vi "Read Joystick.vi"   [LabVIEW 2020]
uses:
  <vilib>/Rock Robotics/WPI/Utilities/WPI_GetSetVariantRefNum.vi
  <vilib>/Rock Robotics/Network Tables/NT Write Boolean Array.vi
  <vilib>/Rock Robotics/Network Tables/NT Write Numeric Array.vi
  Robot Global Data.vi
types:
  T1 = typedef "WPI_JoystickDevRef.ctl" = cluster{"Device":T2}
  T2 = typedef "WPI_JoystickDeviceEnum.ctl" = enum16{"USB 0", "USB 1", "USB 2", "USB 3", "USB 4", "USB 5"}
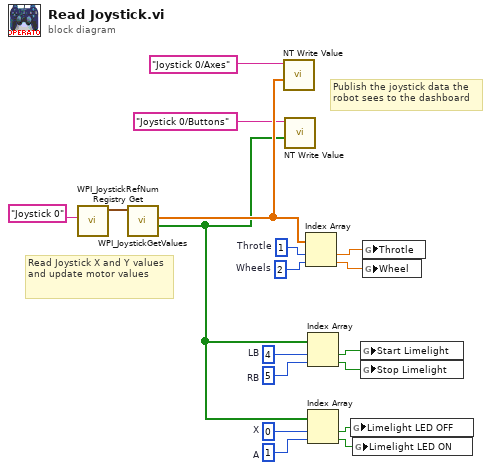
[diagram p0: block diagram]
diagram:
  w3 = 1  # A
  w2 = 0  # X
  w8 = 5  # RB
  w18 = 4  # LB
  w16 = 2  # Wheels
  w15 = 1  # Throtle
  # "Publish the joystick data the\nrobot sees to the dashboard"
  # "Read Joystick X and Y values and update motor values"
  n1 = call <vilib>:"WPI_JoystickRefNum Registry Get.vi"("refnum name"="Joystick 0") -> ("JoystickDevRef"=w12:T1)  [unwired: 1 in, 9 out]
  n2 = call <vilib>:"WPI_JoystickGetValues.vi"("JoystickDevRef"=w12) -> ("Buttons"=w1:bool[], "Axes"=w17:dbl[])  [unwired: 6 in, 3 out]
  n3 = call-poly <vilib>:"NT Write Value.vi"("Numeric Array"=w17, "Name"="Joystick 0/Axes") -> ()  [unwired: 9 in, 1 out]
  n4 = call-poly <vilib>:"NT Write Value.vi"("Boolean Array"=w1, "Name"="Joystick 0/Buttons") -> ()  [unwired: 9 in, 1 out]
  n5 = Index Array(array=w17, index #1=w15, index #2=w16) -> (element #1=w10:dbl, element #2=w9:dbl)
  n6 = Index Array(array=w1, index #1=w18, index #2=w8) -> (element #1=w7:bool, element #2=w6:bool)
  n7 = Index Array(array=w1, index #1=w2, index #2=w3) -> (element #1=w4:bool, element #2=w5:bool)
  n8 = global write "Robot Global Data.vi" "Limelight LED OFF"(w4) -> ()
  n9 = global write "Robot Global Data.vi" "Limelight LED ON"(w5) -> ()
  n10 = global write "Robot Global Data.vi" "Start Limelight"(w7) -> ()
  n11 = global write "Robot Global Data.vi" "Stop Limelight"(w6) -> ()
  n12 = global write "Robot Global Data.vi" "Throtle"(w10) -> ()
  n13 = global write "Robot Global Data.vi" "Wheel"(w9) -> ()
